vi "band_etiq.vi"(3 "Array de entrada":dbl[][](array[numeric])) -> (0 "Numeric":i32, 1 "size(s)":i32[](array[numeric]))   [LabVIEW 2017]
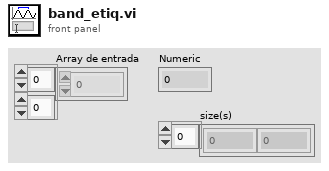
[diagram p1: front panel]
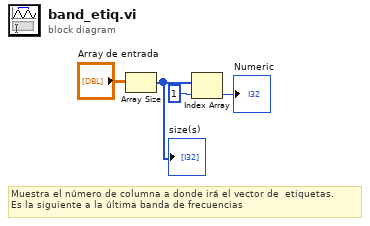
[diagram p0: block diagram]
diagram:
  # "Muestra el número de columna a donde irá el vector de  etiquetas.\nEs la siguiente a la última banda de frecuencias"
  n1 = Array Size(array="Array de entrada") -> (size(s)=w2:i32[])
  "size(s)" <- w2
  n2 = Index Array(array=w2, index=1) -> (element=→"Numeric":i32)
